vi "FPGA_Ready.vi"(7 "Error In":errorcluster, 10 "FPGA VI Reference In":T1) -> (0 "Error Out":errorcluster, 3 "FPGA VI Reference Out":T1)   [LabVIEW 2011]
uses:
  Controls/FPGA SPI_FPGA Ref.ctl
  <vilib>/rvi/interface/nirviReadWriteControl/nirviReadWriteControl.xnode
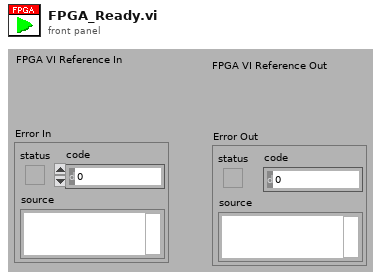
[diagram p1: front panel]
types:
  T1 = typedef "FPGA SPI_FPGA Ref.ctl" = refnum<k20>
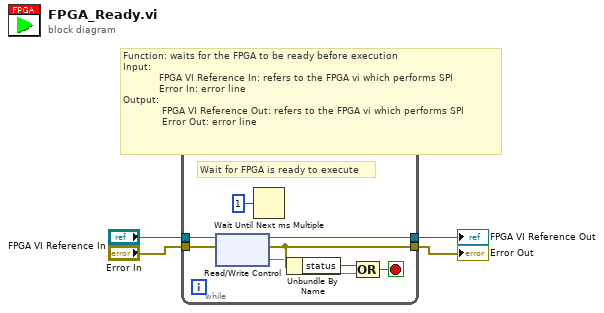
[diagram p0: block diagram]
diagram:
  # "Function: waits for the FPGA to be ready before execution\nInput:\n            FPGA VI Reference In: refers to the FPGA vi which performs SPI\n            Error In: error line\nOutput:\n             FPGA VI Reference Out: refers to the FPGA vi which performs SPI\n             Error Out: error line"
  n1 = while {
    tunnel: "FPGA VI Reference In" -> [w12]
    tunnel: [w11] -> w2
    tunnel: "Error In" -> [w10]
    tunnel: [w8] -> w4
    stop <- w5 stop-if-true
    # "Wait for FPGA is ready to execute"
    n2 = xnode "Read/Write Control"("FPGA VI Reference In"=w12, "error in"=w10) -> ("FPGA VI Reference Out"=w11:T1, "error out"=w8:errorcluster, "Ready"=w6)
    n3 = Wait Until Next ms Multiple(millisecond multiple=u32 1) -> ()  [unwired: 1 out]
    n4 = Unbundle By Name(w8) -> ("status"=w7:bool)
    n5 = Compound Arithmetic op=OR(w7, w6) -> (w5:bool)
  }
  "Error Out" <- w4
  "FPGA VI Reference Out" <- w2
